vi "Recursive Documentation 2012.vi"(8 "error in (no error)":errorcluster, 11 "Project Item Refnum":refnum<vi>) -> (0 "error IO":errorcluster, 3 "String":string)   [LabVIEW 2021]
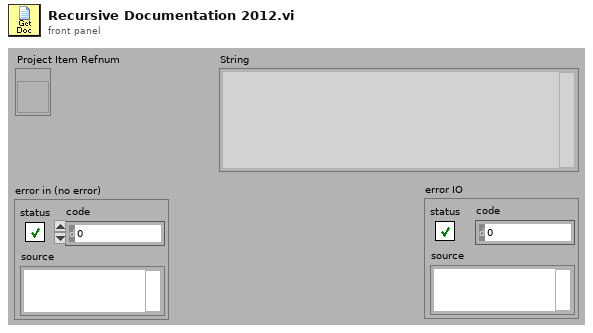
[diagram p1: front panel]
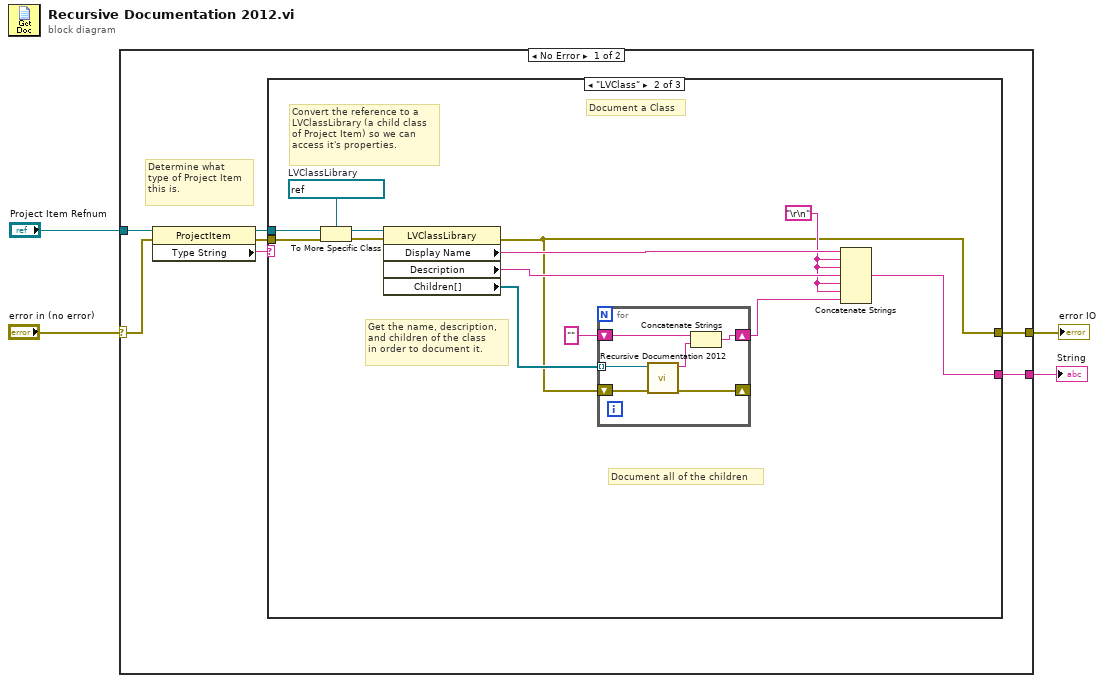
[diagram p0: block diagram]
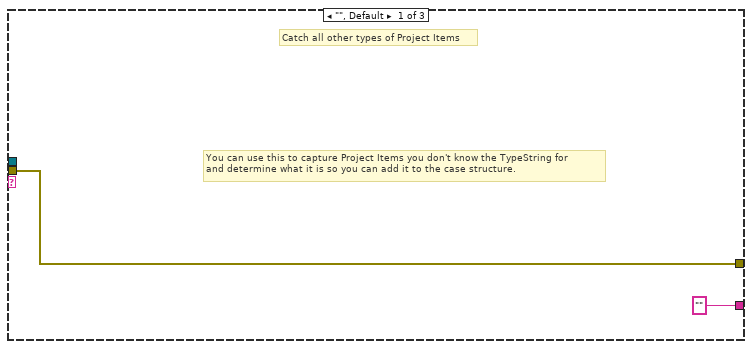
[diagram p2: hidden frame]
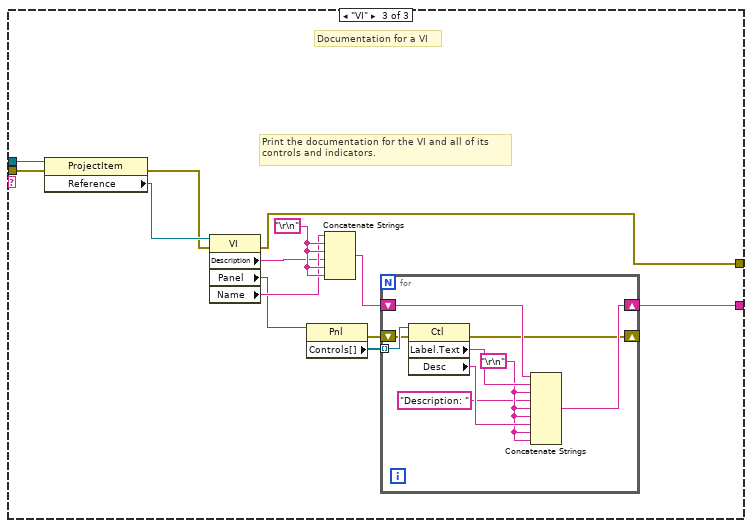
[diagram p3: hidden frame]
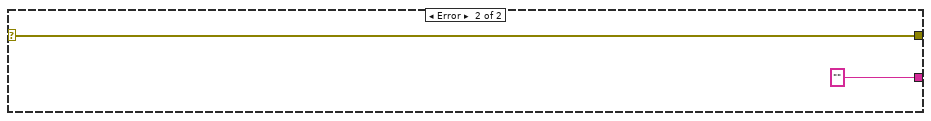
[diagram p4: hidden frame]
diagram:
  n1 = case shown="No Error" "error in (no error)" {
    selector: "error in (no error)" -> [w10 w56]
    tunnel: "Project Item Refnum" -> [w11 _]
    tunnel: [w7 ""] -> w2
    tunnel: [w6 w56] -> w1
    frame No Error {
      # "Determine what\ntype of Project Item\nthis is."
      n2 = property class="ProjectItem"(reference=w11, error in=w10) -> (reference out=w8:refnum<vi>, error out=w5:errorcluster, "Type String"=w9:string)
      n3 = case shown="\"LVClass\"" w9 {
        tunnel: w8 -> [_ w26 w39]
        tunnel: ["" w19 w34] -> w7
        tunnel: [w13 w14 w36] -> w6
        tunnel: w5 -> [w13 w18 w35]
        frame "", Default {
          # "You can use this to capture Project Items you don't know the TypeString for\nand determine what it is so you can add it to the case structure."
          # "Catch all other types of Project Items"
        }
        frame "LVClass" {
          w20 = "\r\n"
          w25 = refnum<vi> refnum  # LVClassLibrary
          # "Document all of the children"
          # "Get the name, description,\nand children of the class\nin order to document it."
          # "Convert the reference to a \nLVClassLibrary (a child class\nof Project Item) so we can\naccess it's properties."
          # "Document a Class"
          n4 = To More Specific Class(target class=w25, reference=w26, error in=w18) -> (specific class reference=w24:refnum<vi>, error out=w23:errorcluster)
          n5 = property class="LVClassLibrary"(reference=w24, error in=w23) -> (error out=w14:errorcluster, "Display Name"=w22:string, "Description"=w21:string, "Children[]"=w17:refnum<vi>[])  [unwired: 1 out]
          n6 = for {
            shift-right: [w31] -> _
            shift-left: w14 -> [w32]
            shift-right: [w28] -> w15
            shift-left: "" -> [w30]
            tunnel: w17 -> [w27] mode=indexing
            n7 = call "Recursive Documentation 2012.vi"("error in (no error)"=w32, "Project Item Refnum"=w27) -> ("error IO"=w31:errorcluster, "String"=w29:string)  [unwired: 8 in]
            n8 = Concatenate Strings(w30, w29) -> (w28:string)
          }
          n9 = Concatenate Strings(w22, w20, w20, w21, w20, w20, w15) -> (w19:string)
        }
        frame "VI" {
          w44 = "\r\n"
          # "Documentation for a VI"
          # "Print the documentation for the VI and all of its\ncontrols and indicators."
          n10 = property class="ProjectItem"(reference=w39, error in=w35) -> (error out=w37:errorcluster, "Reference"=w38:refnum<vi>)  [unwired: 1 out]
          n11 = property class="VI"(reference=w38, error in=w37) -> (error out=w36:errorcluster, "Description"=w42:string, "Panel"=w40:refnum<vi>, "Name"=w43:string)  [unwired: 1 out]
          n12 = property class="Pnl"(reference=w40) -> (error out=w33:errorcluster, "Controls[]"=w41:refnum<vi>[])  [unwired: 1 in, 1 out]
          n13 = Concatenate Strings(w43, w44, w44, w42, w44, w44) -> (w45:string)
          n14 = for {
            tunnel: w41 -> [w54] mode=indexing
            shift-right: [w50] -> w34
            shift-left: w45 -> [w51]
            shift-right: [w46] -> _
            shift-left: w33 -> [w47]
            w49 = "\r\n"
            n15 = property class="Ctl"(reference=w54, error in=w47) -> (error out=w46:errorcluster, "Label.Text"=w53:string, "Desc"=w52:string)  [unwired: 1 out]
            n16 = Concatenate Strings(w51, w53, w49, "Description: " ("string"), w49, w49, w52, w49, w49) -> (w50:string)
          }
        }
      }
    }
    frame Error {
    }
  }
  "String" <- w2
  "error IO" <- w1
